vi "Read Mouse.vi"(8 "error in (no error)":errorcluster, 11 "Refnum in":T1) -> (0 "error out":errorcluster, 1 "Delta y":i16, 2 "Delta x":i16, 3 "Refnum out":T1, 4 "Full packet?":bool, 5 "read buffer":string)   [LabVIEW 2012]
uses:
  FPGA_ref.ctl
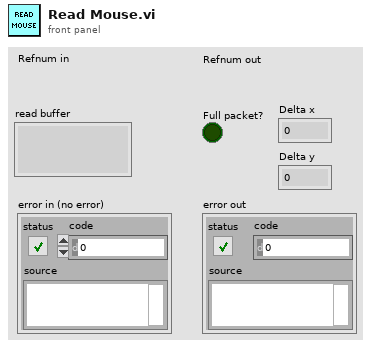
[diagram p1: front panel]
types:
  T1 = typedef "FPGA_ref.ctl" = refnum<k20>
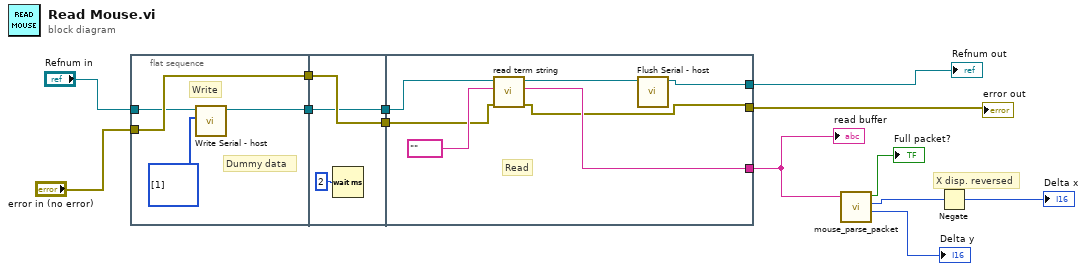
[diagram p0: block diagram]
diagram:
  # "X disp. reversed"
  n1 = flat-sequence {
    tunnel: [w16] -> w13
    tunnel: "error in (no error)" -> [w16]
    tunnel: "Refnum in" -> [w15]
    tunnel: [w14] -> w12
    tunnel: [w20] -> w11
    tunnel: w13 -> [w20]
    tunnel: [w18] -> w10
    tunnel: w12 -> [w18]
    tunnel: [w23] -> w2
    tunnel: [w26] -> w4
    tunnel: w11 -> [w25]
    tunnel: w10 -> [w22]
    tunnel: [w21] -> w8
    frame #0 {
      # "Dummy data"
      # "Write"
      n2 = call "Write Serial - host.vi"("Data"=u8[] [1], "Refnum in"=w15) -> ("Reference Out"=w14:T1)  [unwired: 9 in]
    }
    frame #1 {
      n3 = Wait (ms)(milliseconds to wait=u32 2) -> ()  [unwired: 1 out]
    }
    frame #2 {
      # "Read"
      n4 = call "read term string.vi"("error in (no error)"=w25, "Termination String"="", "Refnum in"=w22) -> ("Error Out"=w23:errorcluster, "Read String"=w26:string, "Reference Out"=w24:T1)  [unwired: 2 in]
      n5 = call "Flush Serial - host.vi"("Refnum in"=w24) -> ("Reference Out"=w21:T1)  [unwired: 10 in]
    }
  }
  n6 = call "mouse_parse_packet.vi"("Data in"=w4) -> ("Full packet?"=→"Full packet?":bool, "Delta x"=w9:i16, "Delta y"=→"Delta y":i16)  [unwired: 3 in]
  n7 = Negate(x=w9) -> (-x=→"Delta x":i16)
  "read buffer" <- w4
  "Refnum out" <- w8
  "error out" <- w2
